vi "배열에 값을 순차적으로 입력하기.vi"() -> ()   [LabVIEW 2014]
panel:
  in  "배열":dbl[](array[numeric])
  out "웨이브폼 차트":dbl[](graph)
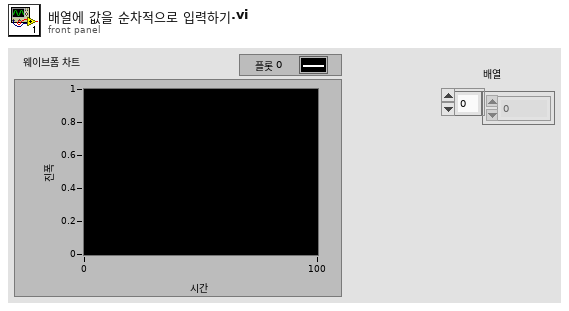
[diagram p1: front panel]
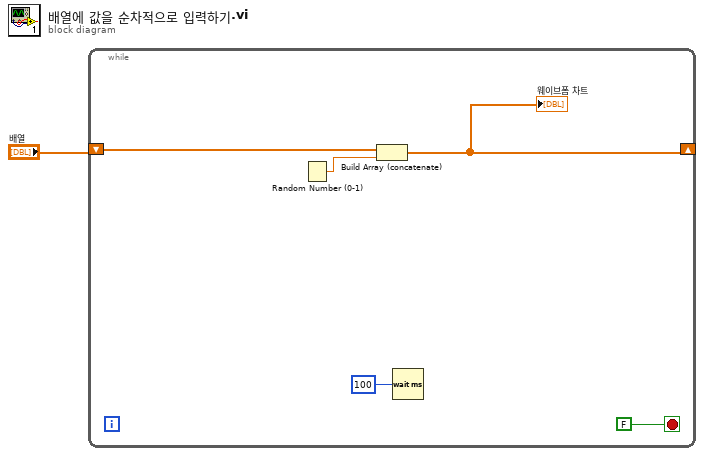
[diagram p0: block diagram]
diagram:
  n1 = while {
    shift-right: [w2] -> _
    shift-left: "배열" -> [w4]
    stop <- FALSE stop-if-true
    n2 = Random Number (0-1)() -> (number: 0 to 1=w3:dbl)
    n3 = Build Array (concatenate)(w4, w3) -> (w2:dbl[])
    "웨이브폼 차트" <- w2
    n4 = Wait (ms)(milliseconds to wait=u32 100 ("대기 시간(ms)")) -> ()  [unwired: 1 out]
  }
